vi "CreateFile (SubVI).vi"(0 "Path name":path, 5 "Save Data":bool, 7 "File name":string, 9 "Date Folder":bool, 11 "error in (no error)":errorcluster, 12 "Add time to file name":bool) -> (4 "Byte Stream File out":refnum<file>, 6 "String":string, 15 "error out":errorcluster)   [LabVIEW 2021]
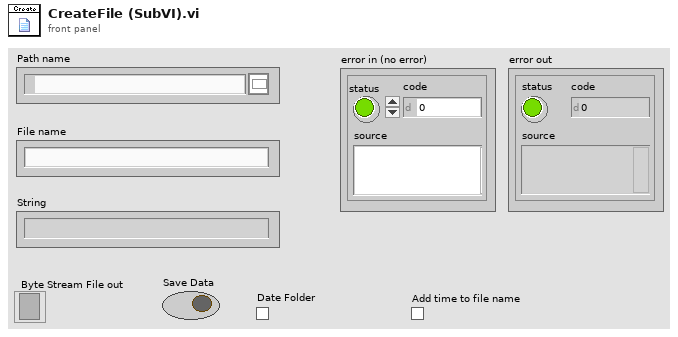
[diagram p1: front panel]
types:
  T1 = enum16{"open", "replace", "create", "open or create", "replace or create", "replace or create with confirmation"}
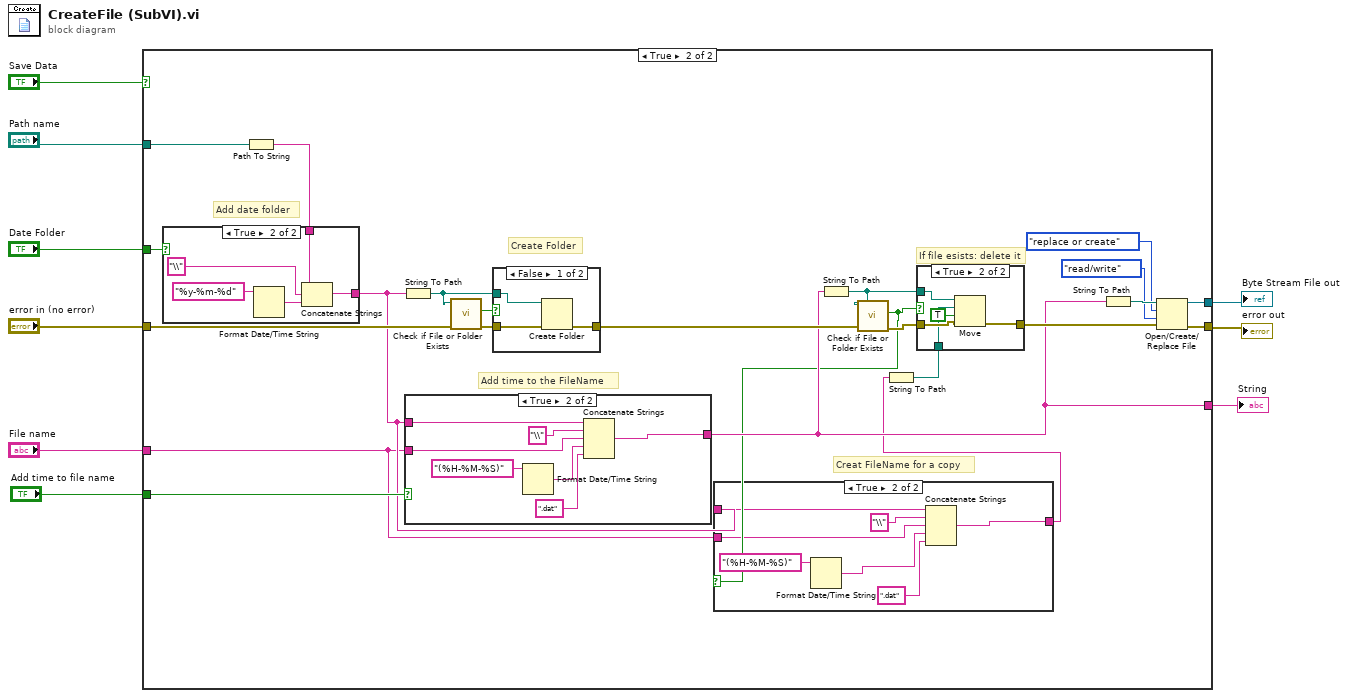
[diagram p0: block diagram]
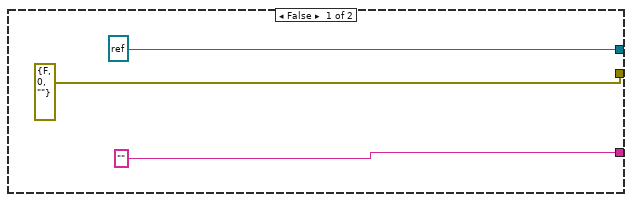
[diagram p2: hidden frame]
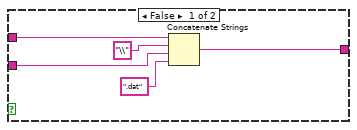
[diagram p3: hidden frame]
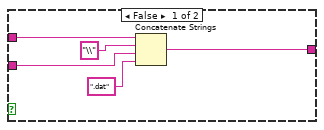
[diagram p4: hidden frame]
diagram:
  n1 = case shown="True" "Save Data" {
    tunnel: [refnum<file> refnum ("refnum out") w35] -> w4
    tunnel: [errorcluster {"status"=FALSE, "code"=0, "source"=""} ("error out") w34] -> w5
    tunnel: "Path name" -> [_ w30]
    tunnel: "File name" -> [_ w16]
    tunnel: ["" w18] -> w9
    tunnel: "error in (no error)" -> [_ w27]
    tunnel: "Date Folder" -> [_ w24]
    tunnel: "Add time to file name" -> [_ w19]
    frame False {
    }
    frame True {
      # "Creat FileName for a copy"
      # "Add time to the FileName"
      # "Add date folder"
      # "If file esists: delete it"
      # "Create Folder"
      n2 = Path To String(path=w30) -> (string=w31:string)
      n3 = case shown="True" w24 {
        tunnel: w31 -> [w66 w68]
        tunnel: [w66 w67] -> w17
        frame False {
        }
        frame True {
          n4 = Format Date/Time String(time format string (%c)="%y-%m-%d") -> (date/time string=w70:string)  [unwired: 2 out]
          n5 = Concatenate Strings(w68, "\\" ("string"), w70) -> (w67:string)
        }
      }
      n6 = String To Path(string=w17) -> (path=w29:path)
      n7 = case shown="True" w19 {
        tunnel: w17 -> [w52 w59]
        tunnel: w16 -> [w50 w53]
        tunnel: [w48 w57] -> w18
        frame False {
          n8 = Concatenate Strings(w52, "\\" ("string"), w50, ".dat" ("string")) -> (w48:string)
        }
        frame True {
          n9 = Format Date/Time String(time format string (%c)="(%H-%M-%S)") -> (date/time string=w54:string)  [unwired: 1 in, 1 out]
          n10 = Concatenate Strings(w59, "\\" ("string"), w53, w54, ".dat" ("string")) -> (w57:string)
        }
      }
      n11 = call <vilib>:"Check if File or Folder Exists.vi"("error in (no error)"=w27, "path"=w29) -> ("error out"=w32:errorcluster, "file or folder exists?"=w33:bool)  [unwired: 7 in, 1 out]
      n12 = case shown="False" w33 {
        tunnel: w32 -> [w74 w75]
        tunnel: [w73 w75] -> w20
        tunnel: w29 -> [w72 _]
        frame False {
          n13 = Create Folder(path (use dialog)=w72, error in=w74) -> (error out=w73:errorcluster)  [unwired: 1 in, 2 out]
        }
        frame True {
        }
      }
      n14 = String To Path(string=w18) -> (path=w22:path)
      n15 = call <vilib>:"Check if File or Folder Exists.vi"("error in (no error)"=w20, "path"=w22) -> ("error out"=w23:errorcluster, "file or folder exists?"=w13:bool)  [unwired: 7 in, 1 out]
      n16 = case shown="True" w13 {
        tunnel: w17 -> [w40 w47]
        tunnel: w16 -> [w38 w45]
        tunnel: [w36 w44] -> w15
        frame False {
          n17 = Concatenate Strings(w40, "\\" ("string"), w38, ".dat" ("string")) -> (w36:string)
        }
        frame True {
          n18 = Format Date/Time String(time format string (%c)="(%H-%M-%S)") -> (date/time string=w41:string)  [unwired: 1 in, 1 out]
          n19 = Concatenate Strings(w47, "\\" ("string"), w45, w41, ".dat" ("string")) -> (w44:string)
        }
      }
      n20 = String To Path(string=w15) -> (path=w14:path)
      n21 = case shown="True" w13 {
        tunnel: w23 -> [w60 w64]
        tunnel: [w60 w65] -> w21
        tunnel: w22 -> [_ w63]
        tunnel: w14 -> [_ w62]
        frame False {
        }
        frame True {
          n22 = Move(source path=w63, error in=w64, 9:TRUE ("overwrite (F)"), 10:w62) -> (error out=w65:errorcluster)  [unwired: 1 in, 2 out]
        }
      }
      n23 = String To Path(string=w18) -> (path=w28:path)
      n24 = Open/Create/Replace File(file path (use dialog)=w28, error in=w21, operation (0:open)=T1."replace or create", access (0:read/write)=enum16{"read/write", "read-only", "write-only"}."read/write") -> (refnum out=w35:refnum<file>, error out=w34:errorcluster)  [unwired: 2 in, 1 out]
    }
  }
  "String" <- w9
  "error out" <- w5
  "Byte Stream File out" <- w4
